vi "20221126_sequence_loader.vi"(0 "Instruct Data":i32[](array[numeric]), 1 "Path":path=path "C:/SpinCore/SpinAPI/lib/spinapi64.dll", 5 "Op Code":i32[](array[numeric]), 7 "Flags":bool[][](array[boolean]), 9 "Comments":string[](array[string]), 11 "Time":dbl[](array[numeric]) format="%#_6p") -> (4 "path out":path=path "C:/SpinCore/SpinAPI/lib/spinapi64.dll")   [LabVIEW 2015]
panel:
  out "Length check":bool
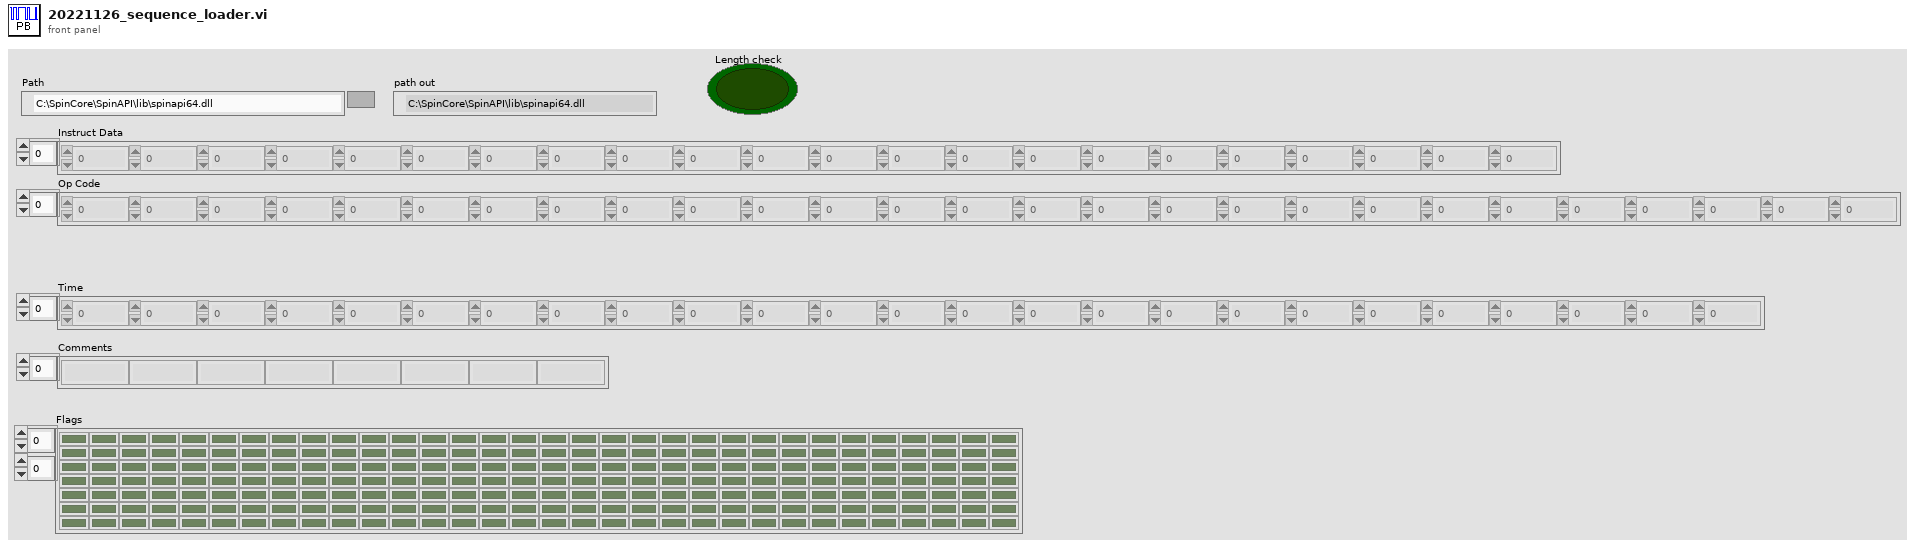
[diagram p1: front panel]
types:
  T1 = enum16{"Pulse Program", "Frequency Registers", "TX Phase Registers", "RX Phase Registers"}
  T2 = cluster{"Numeric":i32, "Numeric":i32, bool[], "String":string, "Numeric":dbl}
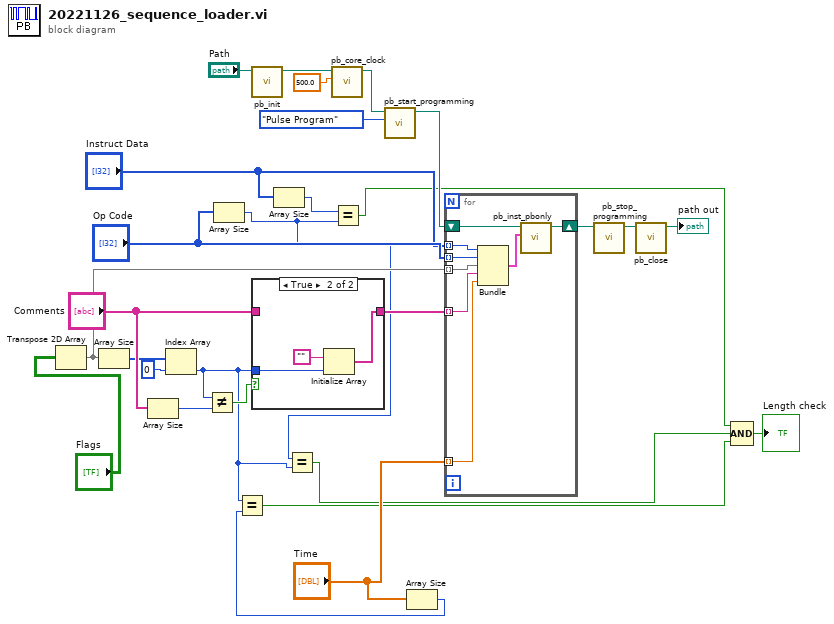
[diagram p0: block diagram]
diagram:
  n1 = Transpose 2D Array(2D array="Flags") -> (transposed array=w13:bool[][])
  n2 = Array Size(array=w13) -> (size(s)=w14:i32[])
  n3 = Array Size(array="Comments") -> (size(s)=w19:i32)
  n4 = Index Array(array=w14, index=0) -> (element=w5:i32)
  n5 = Not Equal?(x=w5, y=w19) -> (x != y?=w18:bool)
  n6 = Array Size(array="Op Code") -> (size(s)=w6:i32)
  n7 = call "pb_init.vi"("path in"="Path") -> ("path out"=w24:path)  [unwired: 9 in, 1 out]
  n8 = case shown="True" w18 {
    tunnel: "Comments" -> [w29 _]
    tunnel: [w29 w30] -> w16
    tunnel: w5 -> [_ w31]
    frame False {
    }
    frame True {
      n9 = Initialize Array("", w31) -> (w30:string[])
    }
  }
  n10 = Array Size(array="Instruct Data") -> (size(s)=w7:i32)
  n11 = Equal?(x=w6, y=w5) -> (x = y?=w3:bool)
  n12 = call "pb_core_clock.vi"("clock_freq (MHz)"=500.0, "path in"=w24) -> ("path out"=w27:path)  [unwired: 8 in, 1 out]
  n13 = Equal?(x=w7, y=w6) -> (x = y?=w2:bool)
  n14 = call "pb_start_programming.vi"("Device"=T1."Pulse Program", "path in"=w27) -> ("path out"=w21:path)  [unwired: 8 in, 1 out]
  n15 = Array Size(array="Time") -> (size(s)=w8:i32)
  n16 = Equal?(x=w5, y=w8) -> (x = y?=w4:bool)
  n17 = for {
    tunnel: "Time" -> [w40] mode=indexing
    tunnel: w16 -> [w39] mode=indexing
    tunnel: w13 -> [w33] mode=indexing
    tunnel: "Op Code" -> [w38] mode=indexing
    tunnel: "Instruct Data" -> [w37] mode=indexing
    shift-right: [w34] -> w20
    shift-left: w21 -> [w35]
    n18 = Bundle("Numeric"=w37, "Numeric"=w38, w33, "String"=w39, "Numeric"=w40) -> (w36:T2)  [unwired: 1 in]
    n19 = call "pb_inst_pbonly.vi"("PB Instruction"=w36, "path in"=w35) -> ("path out"=w34:path)  [unwired: 8 in, 1 out]
  }
  n20 = call "pb_stop_programming.vi"("path in"=w20) -> ("path out"=w22:path)  [unwired: 9 in, 1 out]
  n21 = call "pb_close.vi"("path in"=w22) -> ("path out"=→"path out":path)  [unwired: 9 in, 1 out]
  n22 = Compound Arithmetic op=AND(w2, w3, w4) -> (→"Length check":bool)
